vi "compressFiles-Demo.vi"(0 "mis原始sn字符串":string, 1 "P/N:":string, 2 "NetPathCompress1":path, 3 "NetPathCompress2":path, 4 "NetCmdCompress":string, 5 "original Path":path=path "S:/PNA_Data/L7KQF001-SD-R/SN-152440002_150901", 7 "EEPROMTF":bool=TRUE, 9 "Excel?":bool=TRUE, 11 "db_VNA":string="L7KQF003-SD-R1;l7kqf003-sd-r1510090002;", 12 "S/N:":string="152860001", 13 "条码输出":string) -> ()   [LabVIEW 2011]
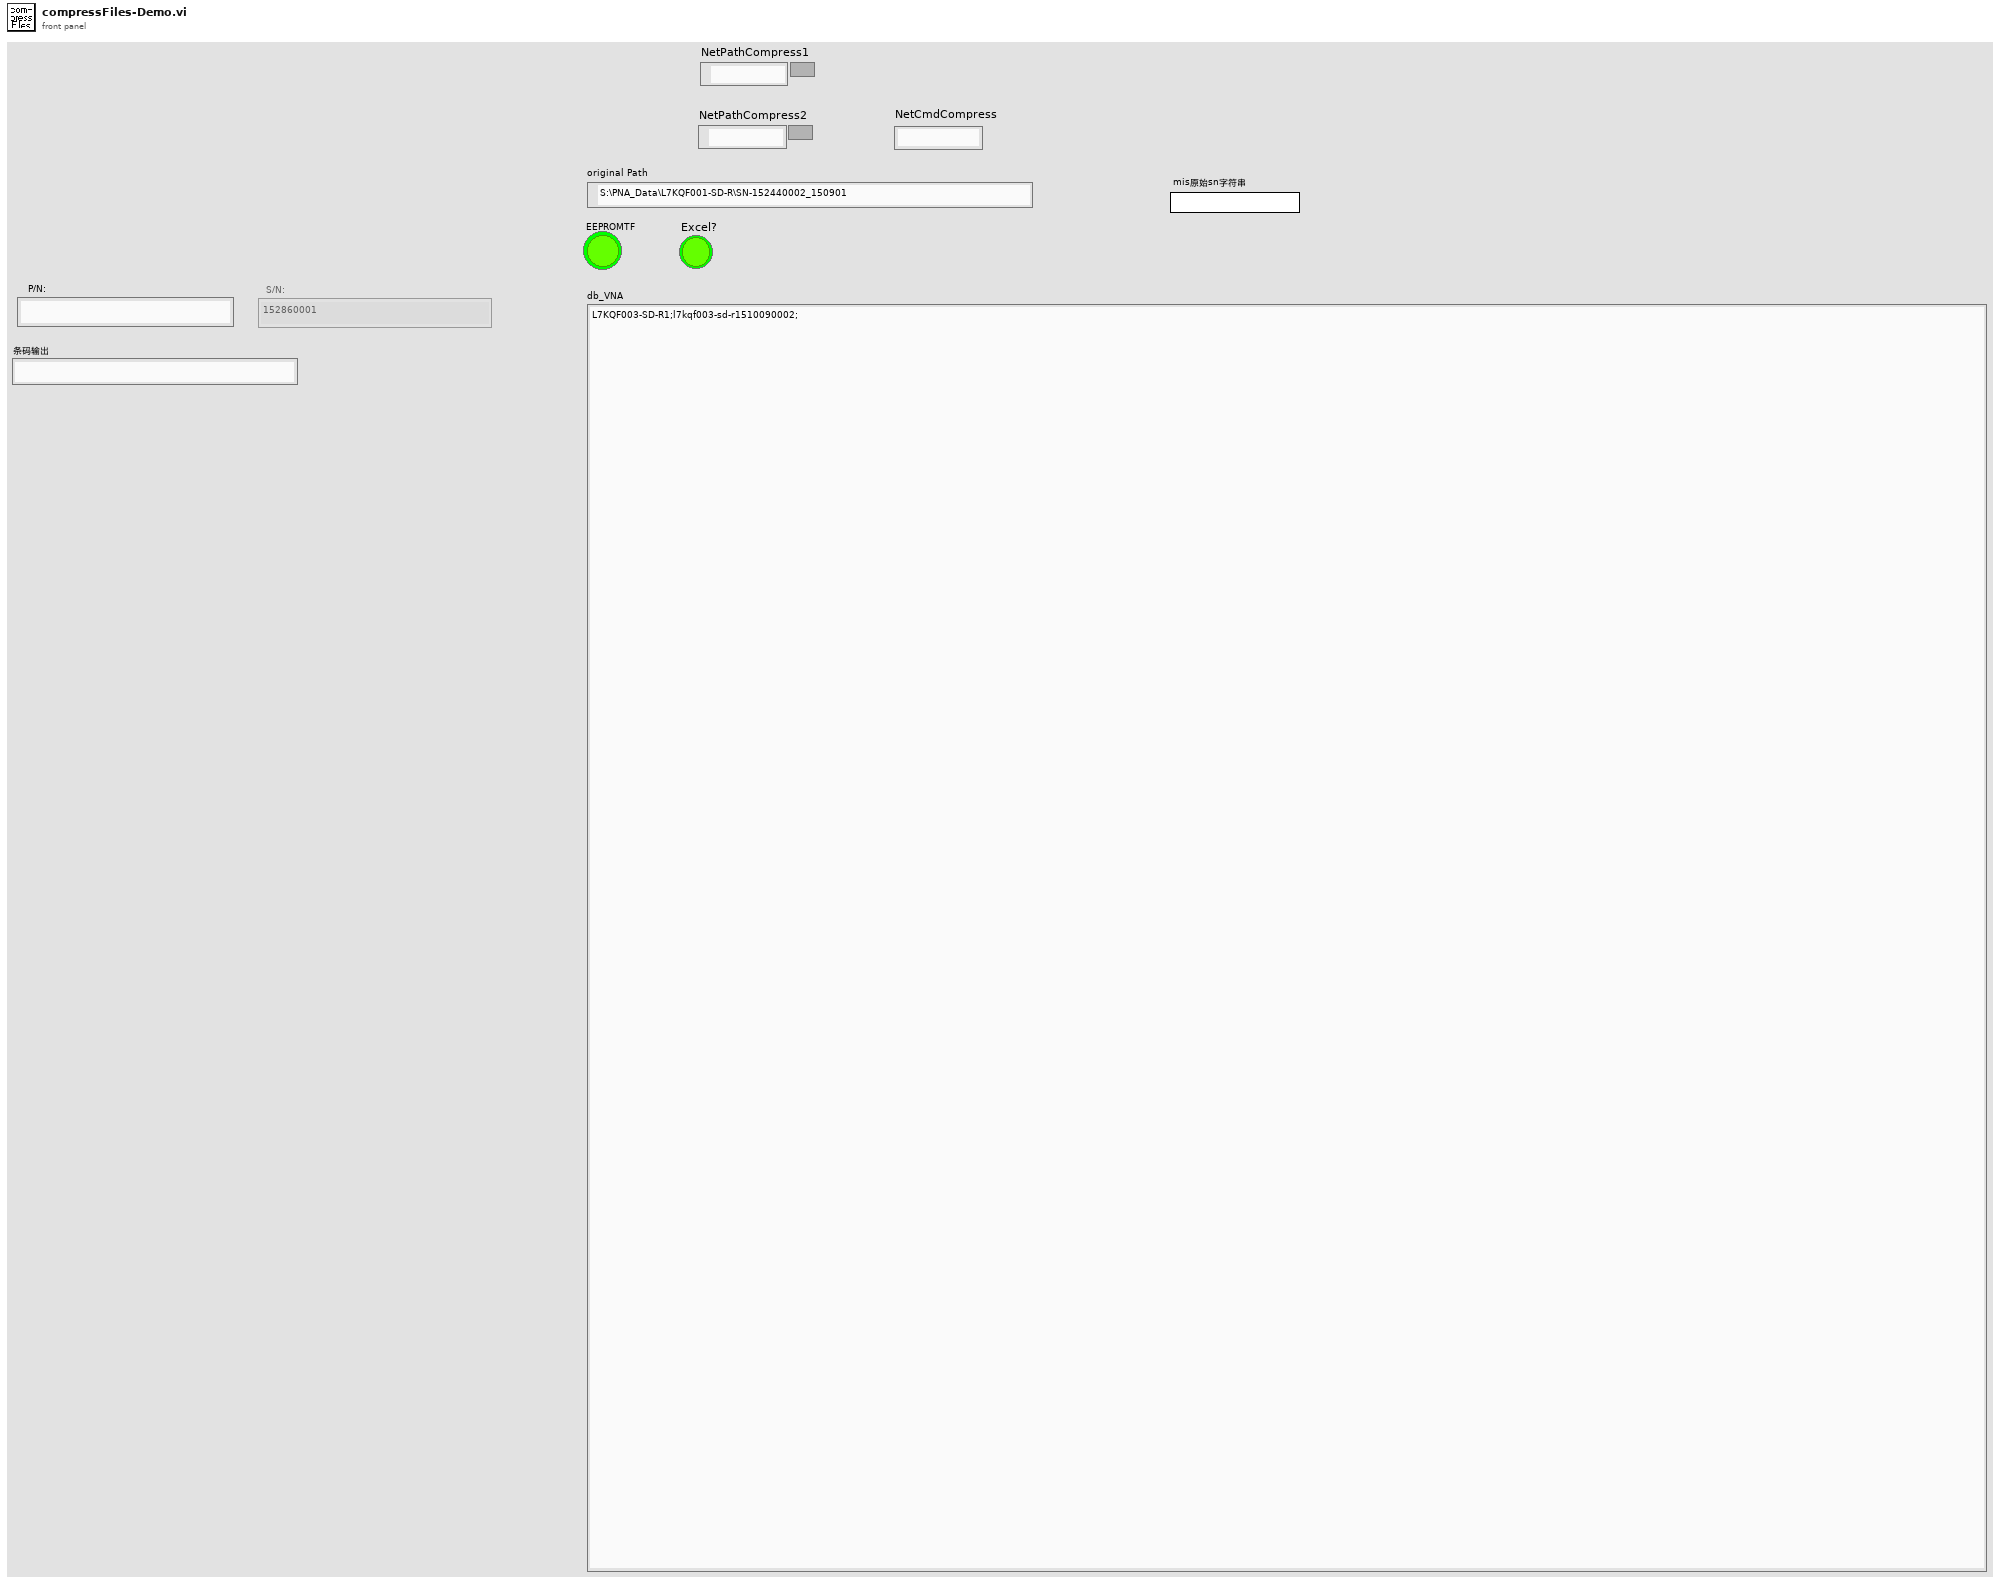
[diagram p1: front panel]
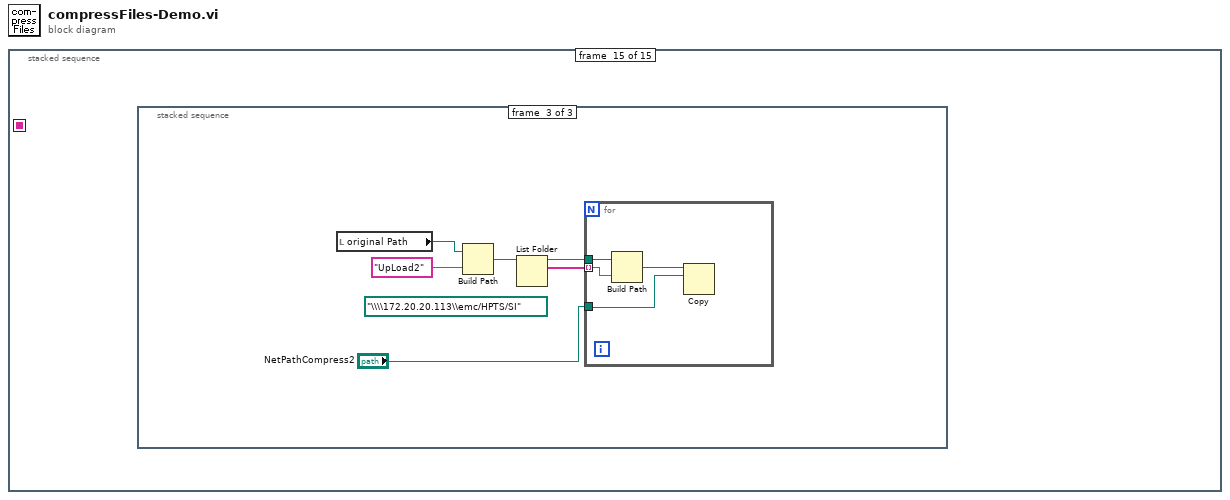
[diagram p0: block diagram]
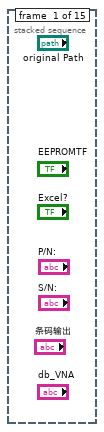
[diagram p2: hidden frame]
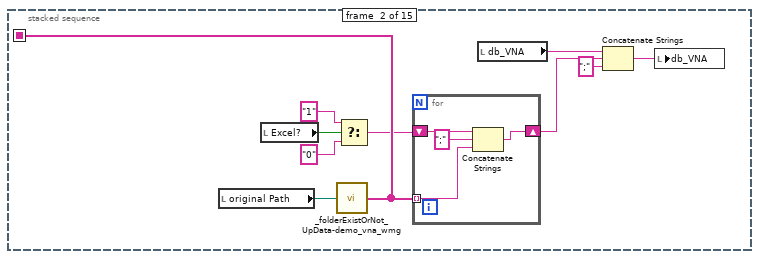
[diagram p3: hidden frame]
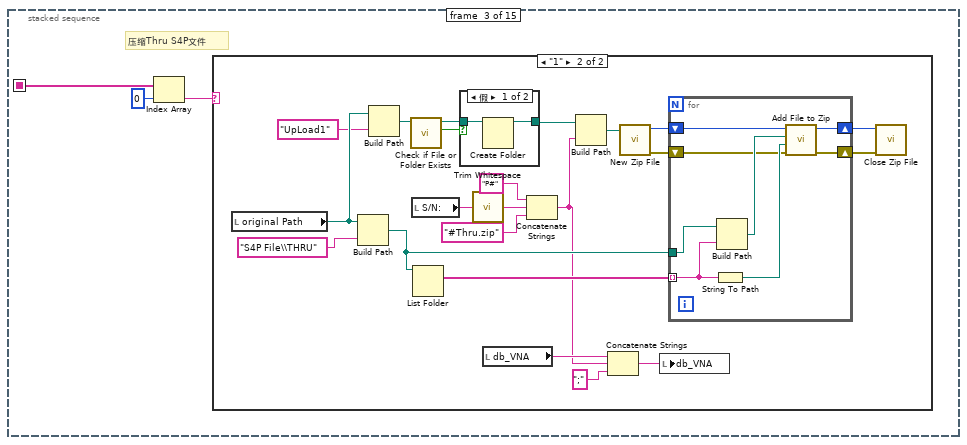
[diagram p4: hidden frame]
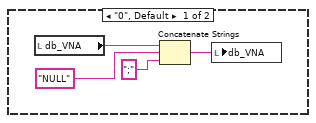
[diagram p5: hidden frame]
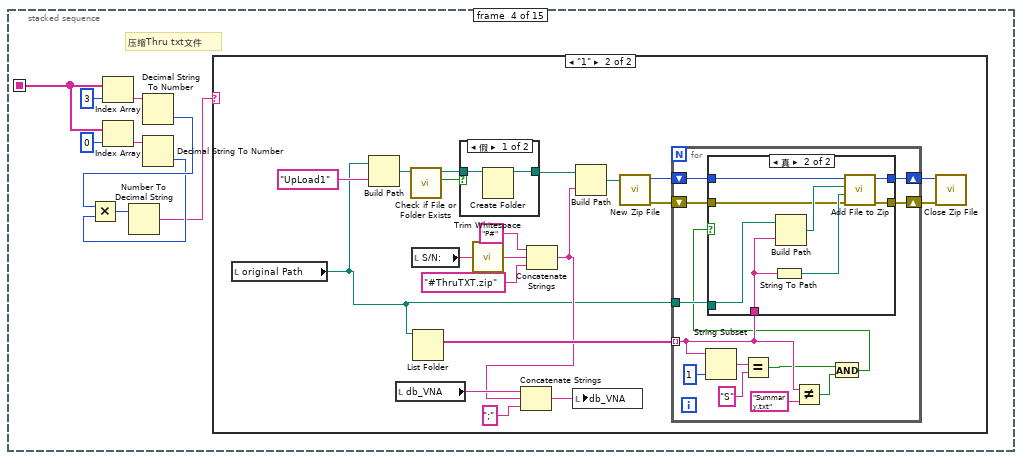
[diagram p7: hidden frame]
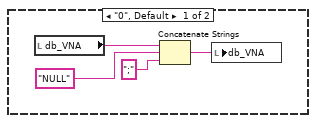
[diagram p8: hidden frame]
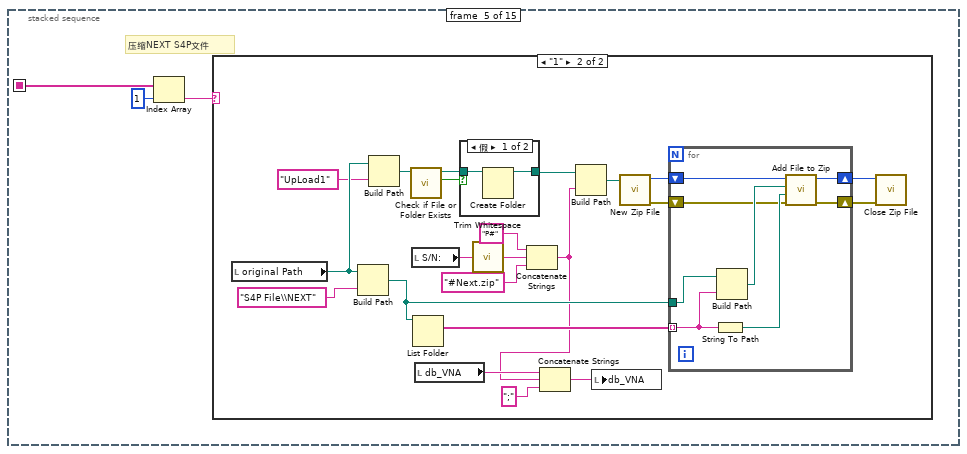
[diagram p11: hidden frame]
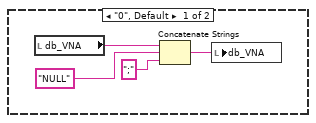
[diagram p12: hidden frame]
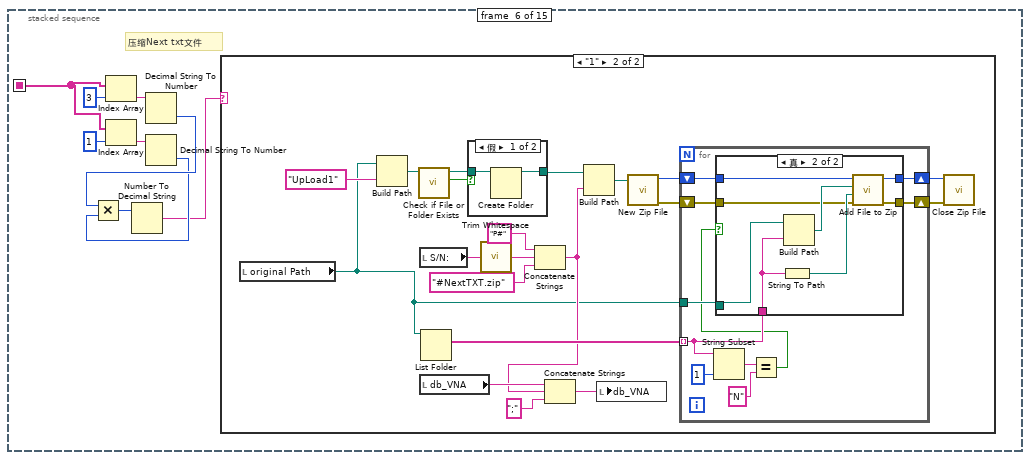
[diagram p14: hidden frame]
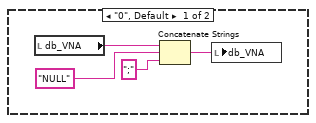
[diagram p15: hidden frame]
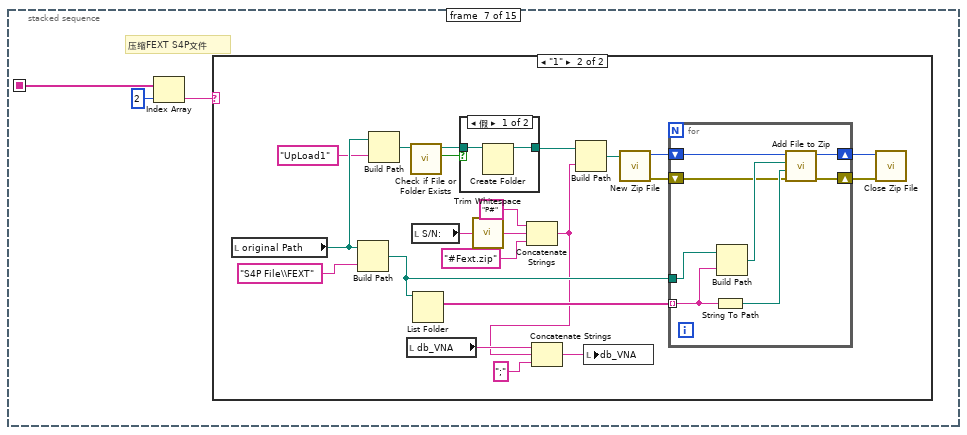
[diagram p18: hidden frame]
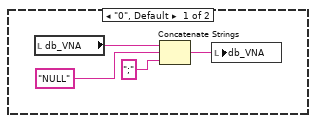
[diagram p19: hidden frame]
diagram:
  n1 = stacked-sequence {
    seq-local: [_ w2 _ _ _ _ _ _ _ _ _ _ _ _ _] -> [_ _ w17 w61 w116 w155 w212 w251 w308 w363 _ w463 _ _ _]
    frame #0 {
    }
    frame #1 {
      n2 = local read "original Path"() -> (w3:path)
      n3 = local read "Excel?"() -> (w10:bool)
      n4 = call "_folderExistOrNot_UpData-demo_vna_wmg.vi"("基础路径"=w3) -> ("output"=w2:string[])
      n5 = Select(t="1", s=w10, f="0") -> (s? t:f=w1:string)
      n6 = for {
        tunnel: w2 -> [w12] mode=indexing
        shift-right: [w11] -> w5
        shift-left: w1 -> [w14]
        n7 = Concatenate Strings(w14, ";" ("字符串"), w12) -> (w11:string)
      }
      n8 = local read "db_VNA"() -> (w7:string)
      n9 = Concatenate Strings(w7, w5, ";" ("字符串")) -> (w6:string)
      n10 = local write "db_VNA"(w6) -> ()
    }
    frame #2 {
      # "压缩Thru S4P文件"
      n11 = Index Array(array=w17, index=0 ("索引")) -> (element=w15:string)
      n12 = case shown="\"1\"" w15 {
        frame "0", Default {
          n13 = local read "db_VNA"() -> (w21:string)
          n14 = Concatenate Strings(w21, "NULL", ";" ("字符串")) -> (w20:string)
          n15 = local write "db_VNA"(w20) -> ()
        }
        frame "1" {
          n16 = local read "original Path"() -> (w42:path)
          n17 = Build Path(base path=w42, name or relative path="S4P File\\THRU") -> (appended path=w31:path)
          n18 = Build Path(base path=w42, name or relative path="UpLoad1" ("名称或相对路径")) -> (appended path=w40:path)
          n19 = call <vilib>:"Check if File or Folder Exists.vi"("path"=w40) -> ("file or folder exists?"=w39:bool, "dup path"=w38:path)  [unwired: 8 in, 1 out]
          n20 = local read "S/N:"() -> (w37:string)
          n21 = List Folder(path=w31) -> (filenames=w32:string[])  [unwired: 3 in, 3 out]
          n22 = case shown="假" w39 {
            tunnel: w38 -> [w53 w54]
            tunnel: [w52 w54] -> w33
            frame False {
              n23 = Create Folder(path (use dialog)=w53) -> (created path=w52:path)  [unwired: 2 in, 2 out]
            }
            frame True {
            }
          }
          n24 = call <vilib>:"Trim Whitespace.vi"("string"=w37) -> ("trimmed string"=w36:string)  [unwired: 1 in]
          n25 = local read "db_VNA"() -> (w25:string)
          n26 = Concatenate Strings("P#", w36, "#Thru.zip") -> (w22:string)
          n27 = Build Path(base path=w33, name or relative path=w22) -> (appended path=w30:path)
          n28 = Concatenate Strings(w25, w22, ";" ("字符串")) -> (w24:string)
          n29 = call <vilib>:"New Zip File.vi"("target"=w30) -> ("error out"=w27:errorcluster, "zip file out"=w29:i64)  [unwired: 4 in, 1 out]
          n30 = local write "db_VNA"(w24) -> ()
          n31 = for {
            tunnel: w32 -> [w50] mode=indexing
            tunnel: w31 -> [w51]
            shift-right: [w48] -> w28
            shift-left: w29 -> [w49]
            shift-right: [w44] -> w26
            shift-left: w27 -> [w45]
            n32 = String To Path(string=w50) -> (path=w46:path)
            n33 = Build Path(base path=w51, name or relative path=w50) -> (appended path=w47:path)
            n34 = call <vilib>:"Add File to Zip.vi"("error in (no error)"=w45, "destination path in zip"=w46, "source file path"=w47, "zip file in"=w49) -> ("error out"=w44:errorcluster, "zip file out"=w48:i64)  [unwired: 6 in]
          }
          n35 = call <vilib>:"Close Zip File.vi"("error in (no error)"=w26, "zip file in"=w28) -> ()  [unwired: 5 in, 1 out]
        }
      }
    }
    frame #3 {
      # "压缩Thru txt文件"
      n36 = Index Array(array=w61, index=3 ("索引")) -> (element=w60:string)
      n37 = Index Array(array=w61, index=0 ("索引")) -> (element=w59:string)
      n38 = Decimal String To Number(string=w60) -> (number=w58:i32)  [unwired: 2 in, 1 out]
      n39 = Decimal String To Number(string=w59) -> (number=w57:i32)  [unwired: 2 in, 1 out]
      n40 = Multiply(x=w58, y=w57) -> (x*y=w56:i32)
      n41 = Number To Decimal String(number=w56) -> (decimal integer string=w55:string)  [unwired: 1 in]
      n42 = case shown="\"1\"" w55 {
        frame "0", Default {
          n43 = local read "db_VNA"() -> (w67:string)
          n44 = Concatenate Strings(w67, "NULL", ";" ("字符串")) -> (w66:string)
          n45 = local write "db_VNA"(w66) -> ()
        }
        frame "1" {
          n46 = local read "original Path"() -> (w68:path)
          n47 = Build Path(base path=w68, name or relative path="UpLoad1" ("名称或相对路径")) -> (appended path=w86:path)
          n48 = local read "db_VNA"() -> (w72:string)
          n49 = call <vilib>:"Check if File or Folder Exists.vi"("path"=w86) -> ("file or folder exists?"=w85:bool, "dup path"=w84:path)  [unwired: 8 in, 1 out]
          n50 = local read "S/N:"() -> (w83:string)
          n51 = List Folder(path=w68) -> (filenames=w78:string[])  [unwired: 3 in, 3 out]
          n52 = case shown="假" w85 {
            tunnel: w84 -> [w112 w113]
            tunnel: [w111 w113] -> w79
            frame False {
              n53 = Create Folder(path (use dialog)=w112) -> (created path=w111:path)  [unwired: 2 in, 2 out]
            }
            frame True {
            }
          }
          n54 = call <vilib>:"Trim Whitespace.vi"("string"=w83) -> ("trimmed string"=w82:string)  [unwired: 1 in]
          n55 = Concatenate Strings("P#", w82, "#ThruTXT.zip") -> (w69:string)
          n56 = Concatenate Strings(w72, w69, ";" ("字符串")) -> (w71:string)
          n57 = local write "db_VNA"(w71) -> ()
          n58 = Build Path(base path=w79, name or relative path=w69) -> (appended path=w77:path)
          n59 = call <vilib>:"New Zip File.vi"("target"=w77) -> ("error out"=w74:errorcluster, "zip file out"=w76:i64)  [unwired: 4 in, 1 out]
          n60 = for {
            tunnel: w78 -> [w92] mode=indexing
            tunnel: w68 -> [w100]
            shift-right: [w98] -> w75
            shift-left: w76 -> [w99]
            shift-right: [w96] -> w73
            shift-left: w74 -> [w97]
            n61 = String Subset(string=w92, length (rest)=1 ("长度（剩余）")) -> (substring=w94:string)  [unwired: 1 in]
            n62 = Equal?(x=w94, y="S") -> (x = y?=w89:bool)
            n63 = Not Equal?(x=w92, y="Summary.txt") -> (x != y?=w90:bool)
            n64 = And(x=w89, y=w90) -> (x .and. y?=w88:bool)
            n65 = case shown="真" w88 {
              tunnel: w100 -> [_ w110]
              tunnel: w99 -> [w102 w109]
              tunnel: [w102 w108] -> w98
              tunnel: w97 -> [w101 w105]
              tunnel: [w101 w104] -> w96
              tunnel: w92 -> [_ w103]
              frame False {
              }
              frame True {
                n66 = String To Path(string=w103) -> (path=w106:path)
                n67 = Build Path(base path=w110, name or relative path=w103) -> (appended path=w107:path)
                n68 = call <vilib>:"Add File to Zip.vi"("error in (no error)"=w105, "destination path in zip"=w106, "source file path"=w107, "zip file in"=w109) -> ("error out"=w104:errorcluster, "zip file out"=w108:i64)  [unwired: 6 in]
              }
            }
          }
          n69 = call <vilib>:"Close Zip File.vi"("error in (no error)"=w73, "zip file in"=w75) -> ()  [unwired: 5 in, 1 out]
        }
      }
    }
    frame #4 {
      # "压缩NEXT S4P文件"
      n70 = Index Array(array=w116, index=1 ("索引")) -> (element=w114:string)
      n71 = case shown="\"1\"" w114 {
        frame "0", Default {
          n72 = local read "db_VNA"() -> (w120:string)
          n73 = Concatenate Strings(w120, "NULL", ";" ("字符串")) -> (w119:string)
          n74 = local write "db_VNA"(w119) -> ()
        }
        frame "1" {
          n75 = local read "original Path"() -> (w141:path)
          n76 = Build Path(base path=w141, name or relative path="S4P File\\NEXT") -> (appended path=w130:path)
          n77 = Build Path(base path=w141, name or relative path="UpLoad1" ("名称或相对路径")) -> (appended path=w139:path)
          n78 = call <vilib>:"Check if File or Folder Exists.vi"("path"=w139) -> ("file or folder exists?"=w138:bool, "dup path"=w137:path)  [unwired: 8 in, 1 out]
          n79 = local read "S/N:"() -> (w136:string)
          n80 = List Folder(path=w130) -> (filenames=w131:string[])  [unwired: 3 in, 3 out]
          n81 = local read "db_VNA"() -> (w122:string)
          n82 = case shown="假" w138 {
            tunnel: w137 -> [w152 w153]
            tunnel: [w151 w153] -> w132
            frame False {
              n83 = Create Folder(path (use dialog)=w152) -> (created path=w151:path)  [unwired: 2 in, 2 out]
            }
            frame True {
            }
          }
          n84 = call <vilib>:"Trim Whitespace.vi"("string"=w136) -> ("trimmed string"=w135:string)  [unwired: 1 in]
          n85 = Concatenate Strings("P#", w135, "#Next.zip") -> (w121:string)
          n86 = Concatenate Strings(w122, w121, ";" ("字符串")) -> (w123:string)
          n87 = Build Path(base path=w132, name or relative path=w121) -> (appended path=w129:path)
          n88 = local write "db_VNA"(w123) -> ()
          n89 = call <vilib>:"New Zip File.vi"("target"=w129) -> ("error out"=w126:errorcluster, "zip file out"=w128:i64)  [unwired: 4 in, 1 out]
          n90 = for {
            tunnel: w131 -> [w149] mode=indexing
            tunnel: w130 -> [w150]
            shift-right: [w147] -> w127
            shift-left: w128 -> [w148]
            shift-right: [w143] -> w125
            shift-left: w126 -> [w144]
            n91 = String To Path(string=w149) -> (path=w145:path)
            n92 = Build Path(base path=w150, name or relative path=w149) -> (appended path=w146:path)
            n93 = call <vilib>:"Add File to Zip.vi"("error in (no error)"=w144, "destination path in zip"=w145, "source file path"=w146, "zip file in"=w148) -> ("error out"=w143:errorcluster, "zip file out"=w147:i64)  [unwired: 6 in]
          }
          n94 = call <vilib>:"Close Zip File.vi"("error in (no error)"=w125, "zip file in"=w127) -> ()  [unwired: 5 in, 1 out]
        }
      }
    }
    frame #5 {
      # "压缩Next txt文件"
      n95 = Index Array(array=w155, index=3 ("索引")) -> (element=w160:string)
      n96 = Index Array(array=w155, index=1 ("索引")) -> (element=w159:string)
      n97 = Decimal String To Number(string=w160) -> (number=w158:i32)  [unwired: 2 in, 1 out]
      n98 = Decimal String To Number(string=w159) -> (number=w157:i32)  [unwired: 2 in, 1 out]
      n99 = Multiply(x=w158, y=w157) -> (x*y=w156:i32)
      n100 = Number To Decimal String(number=w156) -> (decimal integer string=w154:string)  [unwired: 1 in]
      n101 = case shown="\"1\"" w154 {
        frame "0", Default {
          n102 = local read "db_VNA"() -> (w166:string)
          n103 = Concatenate Strings(w166, "NULL", ";" ("字符串")) -> (w165:string)
          n104 = local write "db_VNA"(w165) -> ()
        }
        frame "1" {
          n105 = local read "original Path"() -> (w167:path)
          n106 = Build Path(base path=w167, name or relative path="UpLoad1" ("名称或相对路径")) -> (appended path=w185:path)
          n107 = call <vilib>:"Check if File or Folder Exists.vi"("path"=w185) -> ("file or folder exists?"=w184:bool, "dup path"=w183:path)  [unwired: 8 in, 1 out]
          n108 = local read "S/N:"() -> (w182:string)
          n109 = local read "db_VNA"() -> (w171:string)
          n110 = List Folder(path=w167) -> (filenames=w177:string[])  [unwired: 3 in, 3 out]
          n111 = case shown="假" w184 {
            tunnel: w183 -> [w208 w209]
            tunnel: [w207 w209] -> w178
            frame False {
              n112 = Create Folder(path (use dialog)=w208) -> (created path=w207:path)  [unwired: 2 in, 2 out]
            }
            frame True {
            }
          }
          n113 = call <vilib>:"Trim Whitespace.vi"("string"=w182) -> ("trimmed string"=w181:string)  [unwired: 1 in]
          n114 = Concatenate Strings("P#", w181, "#NextTXT.zip") -> (w168:string)
          n115 = Concatenate Strings(w171, w168, ";" ("字符串")) -> (w170:string)
          n116 = Build Path(base path=w178, name or relative path=w168) -> (appended path=w176:path)
          n117 = local write "db_VNA"(w170) -> ()
          n118 = call <vilib>:"New Zip File.vi"("target"=w176) -> ("error out"=w173:errorcluster, "zip file out"=w175:i64)  [unwired: 4 in, 1 out]
          n119 = for {
            tunnel: w177 -> [w191] mode=indexing
            tunnel: w167 -> [w196]
            shift-right: [w194] -> w174
            shift-left: w175 -> [w195]
            shift-right: [w192] -> w172
            shift-left: w173 -> [w193]
            n120 = String Subset(string=w191, length (rest)=1 ("长度（剩余）")) -> (substring=w189:string)  [unwired: 1 in]
            n121 = Equal?(x=w189, y="N") -> (x = y?=w187:bool)
            n122 = case shown="真" w187 {
              tunnel: w196 -> [_ w206]
              tunnel: w195 -> [w198 w205]
              tunnel: [w198 w204] -> w194
              tunnel: w193 -> [w197 w201]
              tunnel: [w197 w200] -> w192
              tunnel: w191 -> [_ w199]
              frame False {
              }
              frame True {
                n123 = String To Path(string=w199) -> (path=w202:path)
                n124 = Build Path(base path=w206, name or relative path=w199) -> (appended path=w203:path)
                n125 = call <vilib>:"Add File to Zip.vi"("error in (no error)"=w201, "destination path in zip"=w202, "source file path"=w203, "zip file in"=w205) -> ("error out"=w200:errorcluster, "zip file out"=w204:i64)  [unwired: 6 in]
              }
            }
          }
          n126 = call <vilib>:"Close Zip File.vi"("error in (no error)"=w172, "zip file in"=w174) -> ()  [unwired: 5 in, 1 out]
        }
      }
    }
    frame #6 {
      # "压缩FEXT S4P文件"
      n127 = Index Array(array=w212, index=2 ("索引")) -> (element=w210:string)
      n128 = case shown="\"1\"" w210 {
        frame "0", Default {
          n129 = local read "db_VNA"() -> (w216:string)
          n130 = Concatenate Strings(w216, "NULL", ";" ("字符串")) -> (w215:string)
          n131 = local write "db_VNA"(w215) -> ()
        }
        frame "1" {
          n132 = local read "original Path"() -> (w237:path)
          n133 = Build Path(base path=w237, name or relative path="S4P File\\FEXT") -> (appended path=w226:path)
          n134 = Build Path(base path=w237, name or relative path="UpLoad1" ("名称或相对路径")) -> (appended path=w235:path)
          n135 = local read "db_VNA"() -> (w218:string)
          n136 = call <vilib>:"Check if File or Folder Exists.vi"("path"=w235) -> ("file or folder exists?"=w234:bool, "dup path"=w233:path)  [unwired: 8 in, 1 out]
          n137 = local read "S/N:"() -> (w232:string)
          n138 = List Folder(path=w226) -> (filenames=w227:string[])  [unwired: 3 in, 3 out]
          n139 = case shown="假" w234 {
            tunnel: w233 -> [w248 w249]
            tunnel: [w247 w249] -> w228
            frame False {
              n140 = Create Folder(path (use dialog)=w248) -> (created path=w247:path)  [unwired: 2 in, 2 out]
            }
            frame True {
            }
          }
          n141 = call <vilib>:"Trim Whitespace.vi"("string"=w232) -> ("trimmed string"=w231:string)  [unwired: 1 in]
          n142 = Concatenate Strings("P#", w231, "#Fext.zip") -> (w217:string)
          n143 = Concatenate Strings(w218, w217, ";" ("字符串")) -> (w219:string)
          n144 = Build Path(base path=w228, name or relative path=w217) -> (appended path=w225:path)
          n145 = local write "db_VNA"(w219) -> ()
          n146 = call <vilib>:"New Zip File.vi"("target"=w225) -> ("error out"=w222:errorcluster, "zip file out"=w224:i64)  [unwired: 4 in, 1 out]
          n147 = for {
            tunnel: w227 -> [w245] mode=indexing
            tunnel: w226 -> [w246]
            shift-right: [w243] -> w223
            shift-left: w224 -> [w244]
            shift-right: [w239] -> w221
            shift-left: w222 -> [w240]
            n148 = String To Path(string=w245) -> (path=w241:path)
            n149 = Build Path(base path=w246, name or relative path=w245) -> (appended path=w242:path)
            n150 = call <vilib>:"Add File to Zip.vi"("error in (no error)"=w240, "destination path in zip"=w241, "source file path"=w242, "zip file in"=w244) -> ("error out"=w239:errorcluster, "zip file out"=w243:i64)  [unwired: 6 in]
          }
          n151 = call <vilib>:"Close Zip File.vi"("error in (no error)"=w221, "zip file in"=w223) -> ()  [unwired: 5 in, 1 out]
        }
      }
    }
    frame #7 {
      # "压缩Fext txt文件"
      n152 = Index Array(array=w251, index=3 ("索引")) -> (element=w256:string)
      n153 = Index Array(array=w251, index=2 ("索引")) -> (element=w255:string)
      n154 = Decimal String To Number(string=w256) -> (number=w254:i32)  [unwired: 2 in, 1 out]
      n155 = Decimal String To Number(string=w255) -> (number=w253:i32)  [unwired: 2 in, 1 out]
      n156 = Multiply(x=w254, y=w253) -> (x*y=w252:i32)
      n157 = Number To Decimal String(number=w252) -> (decimal integer string=w250:string)  [unwired: 1 in]
      n158 = case shown="\"1\"" w250 {
        frame "0", Default {
          n159 = local read "db_VNA"() -> (w262:string)
          n160 = Concatenate Strings(w262, "NULL", ";" ("字符串")) -> (w261:string)
          n161 = local write "db_VNA"(w261) -> ()
        }
        frame "1" {
          n162 = local read "original Path"() -> (w263:path)
          n163 = Build Path(base path=w263, name or relative path="UpLoad1" ("名称或相对路径")) -> (appended path=w281:path)
          n164 = local read "db_VNA"() -> (w267:string)
          n165 = call <vilib>:"Check if File or Folder Exists.vi"("path"=w281) -> ("file or folder exists?"=w280:bool, "dup path"=w279:path)  [unwired: 8 in, 1 out]
          n166 = local read "S/N:"() -> (w278:string)
          n167 = List Folder(path=w263) -> (filenames=w273:string[])  [unwired: 3 in, 3 out]
          n168 = case shown="假" w280 {
            tunnel: w279 -> [w304 w305]
            tunnel: [w303 w305] -> w274
            frame False {
              n169 = Create Folder(path (use dialog)=w304) -> (created path=w303:path)  [unwired: 2 in, 2 out]
            }
            frame True {
            }
          }
          n170 = call <vilib>:"Trim Whitespace.vi"("string"=w278) -> ("trimmed string"=w277:string)  [unwired: 1 in]
          n171 = Concatenate Strings("P#", w277, "#FextTXT.zip") -> (w264:string)
          n172 = Concatenate Strings(w267, w264, ";" ("字符串")) -> (w266:string)
          n173 = Build Path(base path=w274, name or relative path=w264) -> (appended path=w272:path)
          n174 = local write "db_VNA"(w266) -> ()
          n175 = call <vilib>:"New Zip File.vi"("target"=w272) -> ("error out"=w269:errorcluster, "zip file out"=w271:i64)  [unwired: 4 in, 1 out]
          n176 = for {
            tunnel: w273 -> [w287] mode=indexing
            tunnel: w263 -> [w292]
            shift-right: [w290] -> w270
            shift-left: w271 -> [w291]
            shift-right: [w288] -> w268
            shift-left: w269 -> [w289]
            n177 = String Subset(string=w287, length (rest)=1 ("长度（剩余）")) -> (substring=w285:string)  [unwired: 1 in]
            n178 = Equal?(x=w285, y="F") -> (x = y?=w283:bool)
            n179 = case shown="真" w283 {
              tunnel: w292 -> [_ w302]
              tunnel: w291 -> [w294 w301]
              tunnel: [w294 w300] -> w290
              tunnel: w289 -> [w293 w297]
              tunnel: [w293 w296] -> w288
              tunnel: w287 -> [_ w295]
              frame False {
              }
              frame True {
                n180 = String To Path(string=w295) -> (path=w298:path)
                n181 = Build Path(base path=w302, name or relative path=w295) -> (appended path=w299:path)
                n182 = call <vilib>:"Add File to Zip.vi"("error in (no error)"=w297, "destination path in zip"=w298, "source file path"=w299, "zip file in"=w301) -> ("error out"=w296:errorcluster, "zip file out"=w300:i64)  [unwired: 6 in]
              }
            }
          }
          n183 = call <vilib>:"Close Zip File.vi"("error in (no error)"=w268, "zip file in"=w270) -> ()  [unwired: 5 in, 1 out]
        }
      }
    }
    frame #8 {
      # "压缩其他 txt文件"
      n184 = Index Array(array=w308, index=3 ("索引")) -> (element=w306:string)
      n185 = case shown="\"1\"" w306 {
        frame "0", Default {
          n186 = local read "db_VNA"() -> (w312:string)
          n187 = Concatenate Strings(w312, "NULL", ";" ("字符串")) -> (w311:string)
          n188 = local write "db_VNA"(w311) -> ()
        }
        frame "1" {
          n189 = local read "original Path"() -> (w313:path)
          n190 = Build Path(base path=w313, name or relative path="UpLoad1" ("名称或相对路径")) -> (appended path=w331:path)
          n191 = local read "db_VNA"() -> (w317:string)
          n192 = call <vilib>:"Check if File or Folder Exists.vi"("path"=w331) -> ("file or folder exists?"=w330:bool, "dup path"=w329:path)  [unwired: 8 in, 1 out]
          n193 = local read "S/N:"() -> (w328:string)
          n194 = List Folder(path=w313) -> (filenames=w323:string[])  [unwired: 3 in, 3 out]
          n195 = case shown="假" w330 {
            tunnel: w329 -> [w359 w360]
            tunnel: [w358 w360] -> w324
            frame False {
              n196 = Create Folder(path (use dialog)=w359) -> (created path=w358:path)  [unwired: 2 in, 2 out]
            }
            frame True {
            }
          }
          n197 = call <vilib>:"Trim Whitespace.vi"("string"=w328) -> ("trimmed string"=w327:string)  [unwired: 1 in]
          n198 = Concatenate Strings("P#", w327, "#TXT.zip") -> (w314:string)
          n199 = Concatenate Strings(w317, w314, ";" ("字符串")) -> (w316:string)
          n200 = local write "db_VNA"(w316) -> ()
          n201 = Build Path(base path=w324, name or relative path=w314) -> (appended path=w322:path)
          n202 = call <vilib>:"New Zip File.vi"("target"=w322) -> ("error out"=w319:errorcluster, "zip file out"=w321:i64)  [unwired: 4 in, 1 out]
          n203 = for {
            tunnel: w323 -> [w342] mode=indexing
            tunnel: w313 -> [w347]
            shift-right: [w345] -> w320
            shift-left: w321 -> [w346]
            shift-right: [w343] -> w318
            shift-left: w319 -> [w344]
            n204 = String Subset(string=w342, length (rest)=1 ("长度（剩余）")) -> (substring=w338:string)  [unwired: 1 in]
            n205 = Not Equal?(x=w338, y="F") -> (x != y?=w334:bool)
            n206 = Not Equal?(x=w338, y="N") -> (x != y?=w336:bool)
            n207 = Not Equal?(x=w338, y="S") -> (x != y?=w335:bool)
            n208 = Compound Arithmetic op=AND(w334, w336, w335) -> (w333:bool)
            n209 = case shown="真" w333 {
              tunnel: w347 -> [_ w357]
              tunnel: w346 -> [w349 w356]
              tunnel: [w349 w355] -> w345
              tunnel: w344 -> [w348 w352]
              tunnel: [w348 w351] -> w343
              tunnel: w342 -> [_ w350]
              frame False {
              }
              frame True {
                n210 = String To Path(string=w350) -> (path=w353:path)
                n211 = Build Path(base path=w357, name or relative path=w350) -> (appended path=w354:path)
                n212 = call <vilib>:"Add File to Zip.vi"("error in (no error)"=w352, "destination path in zip"=w353, "source file path"=w354, "zip file in"=w356) -> ("error out"=w351:errorcluster, "zip file out"=w355:i64)  [unwired: 6 in]
              }
            }
          }
          n213 = call <vilib>:"Close Zip File.vi"("error in (no error)"=w318, "zip file in"=w320) -> ()  [unwired: 5 in, 1 out]
        }
      }
    }
    frame #9 {
      # "压缩PDF文件"
      n214 = Index Array(array=w363, index=5 ("索引")) -> (element=w361:string)
      n215 = case shown="\"1\"" w361 {
        frame "0", Default {
          n216 = local read "db_VNA"() -> (w367:string)
          n217 = Concatenate Strings(w367, "NULL", ";" ("字符串")) -> (w366:string)
          n218 = local write "db_VNA"(w366) -> ()
        }
        frame "1" {
          n219 = local read "original Path"() -> (w372:path)
          n220 = Build Path(base path=w372, name or relative path="UpLoad1" ("名称或相对路径")) -> (appended path=w386:path)
          n221 = local read "db_VNA"() -> (w371:string)
          n222 = call <vilib>:"Check if File or Folder Exists.vi"("path"=w386) -> ("file or folder exists?"=w385:bool, "dup path"=w384:path)  [unwired: 8 in, 1 out]
          n223 = local read "S/N:"() -> (w383:string)
          n224 = List Folder(path=w372) -> (filenames=w378:string[])  [unwired: 3 in, 3 out]
          n225 = case shown="假" w385 {
            tunnel: w384 -> [w412 w413]
            tunnel: [w411 w413] -> w379
            frame False {
              n226 = Create Folder(path (use dialog)=w412) -> (created path=w411:path)  [unwired: 2 in, 2 out]
            }
            frame True {
            }
          }
          n227 = call <vilib>:"Trim Whitespace.vi"("string"=w383) -> ("trimmed string"=w382:string)  [unwired: 1 in]
          n228 = Concatenate Strings("P#", w382, "#PDF.zip") -> (w368:string)
          n229 = Concatenate Strings(w371, w368, ";" ("字符串")) -> (w370:string)
          n230 = Build Path(base path=w379, name or relative path=w368) -> (appended path=w377:path)
          n231 = local write "db_VNA"(w370) -> ()
          n232 = call <vilib>:"New Zip File.vi"("target"=w377) -> ("error out"=w374:errorcluster, "zip file out"=w376:i64)  [unwired: 4 in, 1 out]
          n233 = for {
            tunnel: w378 -> [w393] mode=indexing
            tunnel: w372 -> [w400]
            shift-right: [w398] -> w375
            shift-left: w376 -> [w399]
            shift-right: [w396] -> w373
            shift-left: w374 -> [w397]
            n234 = Search and Replace String(input string=w393, search string=".xls" ("搜索字符串")) -> (number of replacements=w392:i32)  [unwired: 6 in, 3 out]
            n235 = Search and Replace String(input string=w393, search string=".xlsx" ("搜索字符串")) -> (number of replacements=w391:i32)  [unwired: 6 in, 3 out]
            n236 = Greater Than 0?(x=w392) -> (x > 0?=w390:bool)
            n237 = Greater Than 0?(x=w391) -> (x > 0?=w389:bool)
            n238 = Or(x=w390, y=w389) -> (x .or. y?=w388:bool)
            n239 = case shown="真" w388 {
              tunnel: w400 -> [_ w410]
              tunnel: w399 -> [w402 w409]
              tunnel: [w402 w408] -> w398
              tunnel: w397 -> [w401 w405]
              tunnel: [w401 w404] -> w396
              tunnel: w393 -> [_ w403]
              frame False {
              }
              frame True {
                n240 = String To Path(string=w403) -> (path=w406:path)
                n241 = Build Path(base path=w410, name or relative path=w403) -> (appended path=w407:path)
                n242 = call <vilib>:"Add File to Zip.vi"("error in (no error)"=w405, "destination path in zip"=w406, "source file path"=w407, "zip file in"=w409) -> ("error out"=w404:errorcluster, "zip file out"=w408:i64)  [unwired: 6 in]
              }
            }
          }
          n243 = call <vilib>:"Close Zip File.vi"("error in (no error)"=w373, "zip file in"=w375) -> ()  [unwired: 5 in, 1 out]
        }
      }
    }
    frame #10 {
      # "压缩EEPROM文件"
      n244 = local read "EEPROMTF"() -> (w414:bool)
      n245 = case shown="真" w414 {
        frame False {
          n246 = local read "db_VNA"() -> (w418:string)
          n247 = Concatenate Strings(w418, "NULL", ";" ("字符串")) -> (w417:string)
          n248 = local write "db_VNA"(w417) -> ()
        }
        frame True {
          n249 = local read "original Path"() -> (w419:path)
          n250 = Build Path(base path=w419, name or relative path="UpLoad1" ("名称或相对路径")) -> (appended path=w437:path)
          n251 = local read "db_VNA"() -> (w423:string)
          n252 = call <vilib>:"Check if File or Folder Exists.vi"("path"=w437) -> ("file or folder exists?"=w436:bool, "dup path"=w435:path)  [unwired: 8 in, 1 out]
          n253 = local read "S/N:"() -> (w434:string)
          n254 = List Folder(path=w419) -> (filenames=w429:string[])  [unwired: 3 in, 3 out]
          n255 = case shown="假" w436 {
            tunnel: w435 -> [w459 w460]
            tunnel: [w458 w460] -> w430
            frame False {
              n256 = Create Folder(path (use dialog)=w459) -> (created path=w458:path)  [unwired: 2 in, 2 out]
            }
            frame True {
            }
          }
          n257 = call <vilib>:"Trim Whitespace.vi"("string"=w434) -> ("trimmed string"=w433:string)  [unwired: 1 in]
          n258 = Concatenate Strings("P#", w433, "#EEPROM.zip") -> (w420:string)
          n259 = Concatenate Strings(w423, w420, ";" ("字符串")) -> (w422:string)
          n260 = local write "db_VNA"(w422) -> ()
          n261 = Build Path(base path=w430, name or relative path=w420) -> (appended path=w428:path)
          n262 = call <vilib>:"New Zip File.vi"("target"=w428) -> ("error out"=w425:errorcluster, "zip file out"=w427:i64)  [unwired: 4 in, 1 out]
          n263 = for {
            tunnel: w429 -> [w441] mode=indexing
            tunnel: w419 -> [w447]
            shift-right: [w445] -> w426
            shift-left: w427 -> [w446]
            shift-right: [w443] -> w424
            shift-left: w425 -> [w444]
            n264 = Search and Replace String(input string=w441, search string="EEPROM" ("搜索字符串")) -> (number of replacements=w440:i32)  [unwired: 6 in, 3 out]
            n265 = Greater Than 0?(x=w440) -> (x > 0?=w439:bool)
            n266 = case shown="真" w439 {
              tunnel: w447 -> [_ w457]
              tunnel: w446 -> [w449 w456]
              tunnel: [w449 w455] -> w445
              tunnel: w444 -> [w448 w452]
              tunnel: [w448 w451] -> w443
              tunnel: w441 -> [_ w450]
              frame False {
              }
              frame True {
                n267 = String To Path(string=w450) -> (path=w453:path)
                n268 = Build Path(base path=w457, name or relative path=w450) -> (appended path=w454:path)
                n269 = call <vilib>:"Add File to Zip.vi"("error in (no error)"=w452, "destination path in zip"=w453, "source file path"=w454, "zip file in"=w456) -> ("error out"=w451:errorcluster, "zip file out"=w455:i64)  [unwired: 6 in]
              }
            }
          }
          n270 = call <vilib>:"Close Zip File.vi"("error in (no error)"=w424, "zip file in"=w426) -> ()  [unwired: 5 in, 1 out]
        }
      }
    }
    frame #11 {
      # "压缩Suammary 文件"
      n271 = Index Array(array=w463, index=3 ("索引")) -> (element=w461:string)
      n272 = case shown="\"1\"" w461 {
        frame "0", Default {
          n273 = local read "db_VNA"() -> (w467:string)
          n274 = Concatenate Strings(w467, "NULL", ";" ("字符串")) -> (w466:string)
          n275 = local write "db_VNA"(w466) -> ()
        }
        frame "1" {
          n276 = local read "original Path"() -> (w468:path)
          n277 = Build Path(base path=w468, name or relative path="UpLoad1" ("名称或相对路径")) -> (appended path=w485:path)
          n278 = local read "db_VNA"() -> (w471:string)
          n279 = call <vilib>:"Check if File or Folder Exists.vi"("path"=w485) -> ("file or folder exists?"=w484:bool, "dup path"=w483:path)  [unwired: 8 in, 1 out]
          n280 = local read "S/N:"() -> (w482:string)
          n281 = List Folder(path=w468) -> (filenames=w477:string[])  [unwired: 3 in, 3 out]
          n282 = case shown="假" w484 {
            tunnel: w483 -> [w507 w508]
            tunnel: [w506 w508] -> w478
            frame False {
              n283 = Create Folder(path (use dialog)=w507) -> (created path=w506:path)  [unwired: 2 in, 2 out]
            }
            frame True {
            }
          }
          n284 = call <vilib>:"Trim Whitespace.vi"("string"=w482) -> ("trimmed string"=w481:string)  [unwired: 1 in]
          n285 = Concatenate Strings("P#", w481, "#Summary.zip") -> (w469:string)
          n286 = Concatenate Strings(w471, w469) -> (w470:string)
          n287 = Build Path(base path=w478, name or relative path=w469) -> (appended path=w476:path)
          n288 = local write "db_VNA"(w470) -> ()
          n289 = call <vilib>:"New Zip File.vi"("target"=w476) -> ("error out"=w473:errorcluster, "zip file out"=w475:i64)  [unwired: 4 in, 1 out]
          n290 = for {
            tunnel: w477 -> [w490] mode=indexing
            tunnel: w468 -> [w495]
            shift-right: [w493] -> w474
            shift-left: w475 -> [w494]
            shift-right: [w491] -> w472
            shift-left: w473 -> [w492]
            n291 = Search and Replace String(input string=w490, search string="Summary" ("搜索字符串")) -> (number of replacements=w489:i32)  [unwired: 6 in, 3 out]
            n292 = Greater Than 0?(x=w489) -> (x > 0?=w488:bool)
            n293 = case shown="真" w488 {
              tunnel: w495 -> [_ w505]
              tunnel: w494 -> [w497 w504]
              tunnel: [w497 w503] -> w493
              tunnel: w492 -> [w496 w500]
              tunnel: [w496 w499] -> w491
              tunnel: w490 -> [_ w498]
              frame False {
              }
              frame True {
                n294 = String To Path(string=w498) -> (path=w501:path)
                n295 = Build Path(base path=w505, name or relative path=w498) -> (appended path=w502:path)
                n296 = call <vilib>:"Add File to Zip.vi"("error in (no error)"=w500, "destination path in zip"=w501, "source file path"=w502, "zip file in"=w504) -> ("error out"=w499:errorcluster, "zip file out"=w503:i64)  [unwired: 6 in]
              }
            }
          }
          n297 = call <vilib>:"Close Zip File.vi"("error in (no error)"=w472, "zip file in"=w474) -> ()  [unwired: 5 in, 1 out]
        }
      }
    }
    frame #12 {
      # "生成txt的文件"
      n298 = flat-sequence {
        frame #0 {
          w512 = ";" ("搜索字符串/字符(-)")
          n299 = local read "db_VNA"() -> (w514:string)
          n300 = local read "条码输出"() -> (w511:string)
          n301 = Search/Split String(string=w514, search string/char (-)=w512) -> (substring before match=w513:string, match + rest of string=w509:string)  [unwired: 1 in, 1 out]
          n302 = Concatenate Strings(w513, w512, w511, w509) -> (w510:string)
          n303 = local write "db_VNA"(w510) -> ()
        }
        frame #1 {
          n304 = local read "db_VNA"() -> (w516:string)
          n305 = Concatenate Strings(w516, ";" ("搜索字符串/字符(-)"), "mis原始sn字符串") -> (w518:string)
          n306 = local write "db_VNA"(w518) -> ()
        }
        frame #2 {
          n307 = local read "original Path"() -> (w522:path)
          n308 = Build Path(base path=w522, name or relative path="UpLoad1" ("名称或相对路径")) -> (appended path=w530:path)
          n309 = local read "S/N:"() -> (w527:string)
          n310 = call <vilib>:"Check if File or Folder Exists.vi"("path"=w530) -> ("file or folder exists?"=w529:bool, "dup path"=w528:path)  [unwired: 8 in, 1 out]
          n311 = call <vilib>:"Trim Whitespace.vi"("string"=w527) -> ("trimmed string"=w526:string)  [unwired: 1 in]
          n312 = case shown="假" w529 {
            tunnel: w528 -> [w533 w534]
            tunnel: [w532 w534] -> w523
            frame False {
              n313 = Create Folder(path (use dialog)=w533) -> (created path=w532:path)  [unwired: 2 in, 2 out]
            }
            frame True {
            }
          }
          n314 = Concatenate Strings("P#", w526, "#v.txt") -> (w521:string)
          n315 = local read "db_VNA"() -> (w519:string)
          n316 = Build Path(base path=w523, name or relative path=w521) -> (appended path=w520:path)
          n317 = Write to Text File(file (use dialog)=w520, text=w519) -> ()  [unwired: 2 in, 3 out]
        }
      }
    }
    frame #13 {
      n318 = flat-sequence {
        frame #0 {
          w542 = ";"
          n319 = local read "S/N:"() -> (w540:string)
          n320 = call <vilib>:"Trim Whitespace.vi"("string"=w540) -> ("trimmed string"=w539:string)  [unwired: 1 in]
          n321 = local read "original Path"() -> (w550:path)
          n322 = Concatenate Strings("P#", w539, "#s.zip") -> (w536:string)
          n323 = Build Path(base path=w550, name or relative path="UpLoad2" ("名称或相对路径")) -> (appended path=w558:path)
          n324 = call <vilib>:"Check if File or Folder Exists.vi"("path"=w558) -> ("file or folder exists?"=w557:bool, "dup path"=w556:path)  [unwired: 8 in, 1 out]
          n325 = local read "S/N:"() -> (w555:string)
          n326 = local read "P/N:"() -> (w546:string)
          n327 = local read "S/N:"() -> (w545:string)
          n328 = Format Date/Time String(time format string (%c)="%H:%M:%S %Y/%m/%d") -> (date/time string=w543:string)  [unwired: 2 in]
          n329 = case shown="假" w557 {
            tunnel: w556 -> [w561 w562]
            tunnel: [w560 w562] -> w551
            frame False {
              n330 = Create Folder(path (use dialog)=w561) -> (created path=w560:path)  [unwired: 2 in, 2 out]
            }
            frame True {
            }
          }
          n331 = call <vilib>:"Trim Whitespace.vi"("string"=w555) -> ("trimmed string"=w554:string)  [unwired: 1 in]
          n332 = Concatenate Strings("P#", w554, "#s.txt") -> (w549:string)
          n333 = Build Path(base path=w551, name or relative path=w549) -> (appended path=w548:path)
          n334 = Concatenate Strings(w546, w542, w545, w542, "L037407", w542, w543, w542, "PASS", w542, w536) -> (w541:string)
          n335 = Write to Text File(file (use dialog)=w548, text=w541) -> ()  [unwired: 2 in, 3 out]
        }
        frame #1 {
          n336 = local read "S/N:"() -> (w565:string)
          n337 = local read "original Path"() -> (w569:path)
          n338 = call <vilib>:"Trim Whitespace.vi"("string"=w565) -> ("trimmed string"=w566:string)  [unwired: 1 in]
          n339 = Concatenate Strings("UpLoad2\\" ("名称或相对路径"), "P#", w566, "#s.zip") -> (w563:string)
          n340 = Build Path(base path=w569, name or relative path=w563) -> (appended path=w570:path)
          n341 = call <vilib>:"New Zip File.vi"("target"=w570) -> ("zip file out"=w571:i64)  [unwired: 4 in, 2 out]
          n342 = call <vilib>:"Close Zip File.vi"("zip file in"=w571) -> ()  [unwired: 6 in, 1 out]
        }
      }
    }
    frame #14 {
      n343 = stacked-sequence {
        frame #0 {
          n344 = First Call?() -> (First Call?: T/F=w572:bool)
          n345 = case shown="真" w572 {
            frame False {
            }
            frame True {
              (unwired) "net use \\\\172.20.20.113 mesuser /user:mesuser" ("standard input")
              n346 = call <vilib>:"System Exec.vi"("command line"="NetCmdCompress") -> ()  [unwired: 7 in, 4 out]
            }
          }
        }
        frame #1 {
          (unwired) path "\\\\172.20.20.113\\emc/HPTS/VNA" ("目标路径（使用对话框）")
          n347 = local read "original Path"() -> (w578:path)
          n348 = Build Path(base path=w578, name or relative path="UpLoad1" ("名称或相对路径")) -> (appended path=w577:path)
          n349 = List Folder(path=w577) -> (path out=w575:path, filenames=w576:string[])  [unwired: 3 in, 2 out]
          n350 = for {
            tunnel: w576 -> [w582] mode=indexing
            tunnel: w575 -> [w583]
            tunnel: "NetPathCompress1" -> [w580]
            n351 = Build Path(base path=w583, name or relative path=w582) -> (appended path=w581:path)
            n352 = Copy(10:w580, 11:w581) -> ()  [unwired: 3 in, 3 out]
          }
        }
        frame #2 {
          (unwired) path "\\\\172.20.20.113\\emc/HPTS/SI" ("目标路径（使用对话框）")
          n353 = local read "original Path"() -> (w588:path)
          n354 = Build Path(base path=w588, name or relative path="UpLoad2" ("名称或相对路径")) -> (appended path=w587:path)
          n355 = List Folder(path=w587) -> (path out=w585:path, filenames=w586:string[])  [unwired: 3 in, 2 out]
          n356 = for {
            tunnel: w586 -> [w592] mode=indexing
            tunnel: w585 -> [w593]
            tunnel: "NetPathCompress2" -> [w590]
            n357 = Build Path(base path=w593, name or relative path=w592) -> (appended path=w591:path)
            n358 = Copy(10:w590, 11:w591) -> ()  [unwired: 3 in, 3 out]
          }
        }
      }
    }
  }
